vi "Help Queue UI Control.vi"(8 "error In":errorcluster, 11 "CheckPasswordUI.lvclass":refnum<class "CheckPasswordUI.lvclass">) -> (0 "error out":errorcluster)   [LabVIEW 2021, in "CheckPasswordUI.lvclass"]
uses:
  CheckPasswordUI.lvclass
  CheckPasswordUI.lvclass/CheckPasswordUI.ctl
  bc0fb21a-4521-4633-b11b-158f649b6f7e.vi
  <userlib>/John_Lib/Queue_Self/Q-StringToArray_Sushu.vi
  <vilib>/Utility/error.llb/Trim Whitespace.vi
  <userlib>/John_Lib/Queue_Self/Queue_Self.lvlib
panel:
  out "call chain":string[](array[string])
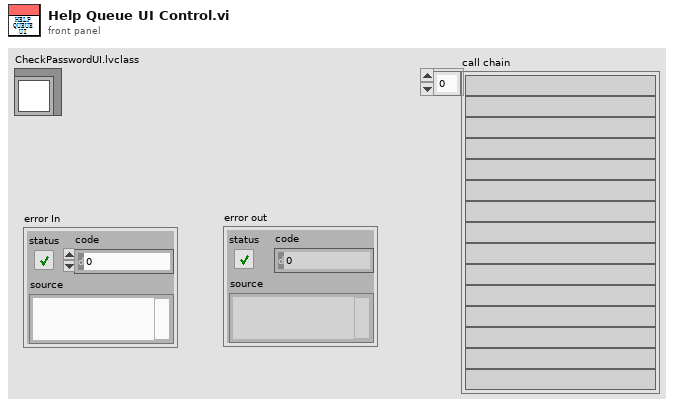
[diagram p1: front panel]
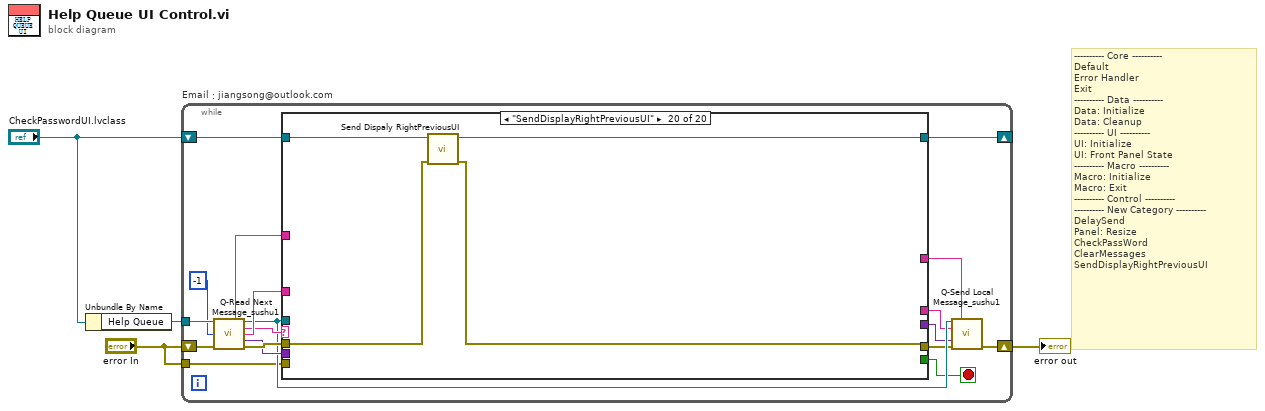
[diagram p0: block diagram]
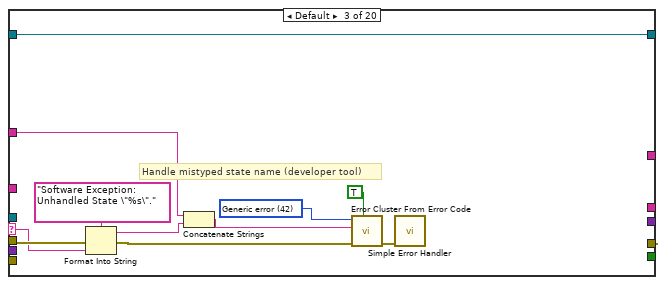
[diagram p4: hidden frame]
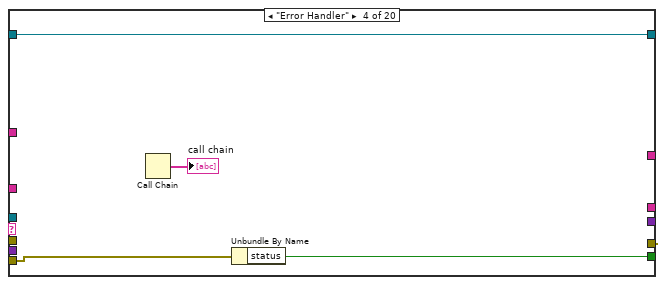
[diagram p5: hidden frame]
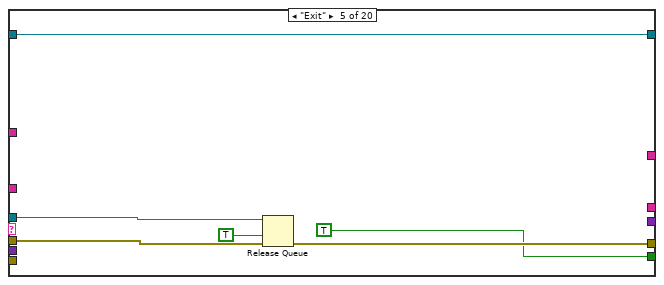
[diagram p6: hidden frame]
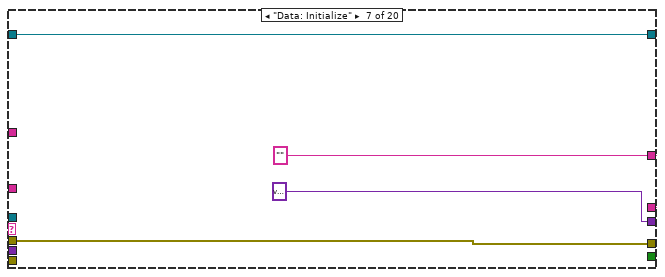
[diagram p8: hidden frame]
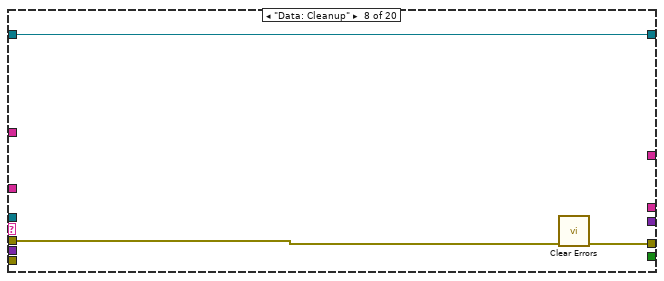
[diagram p9: hidden frame]
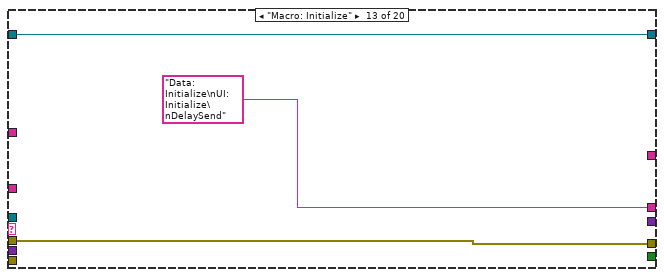
[diagram p14: hidden frame]
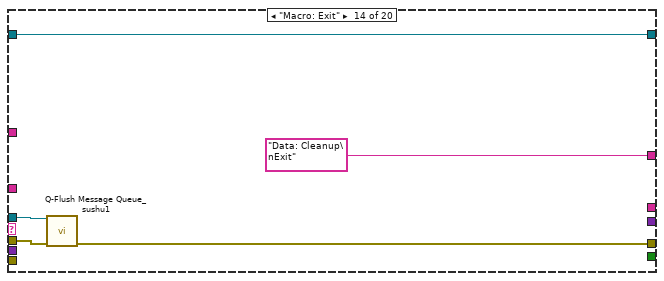
[diagram p15: hidden frame]
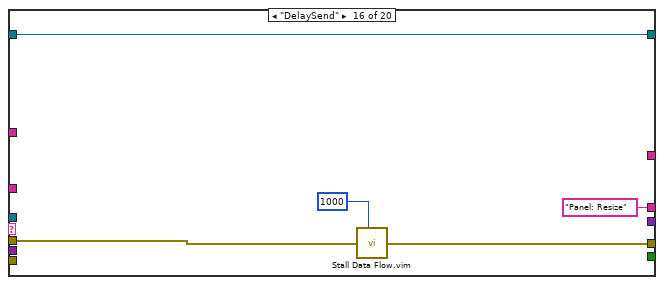
[diagram p17: hidden frame]
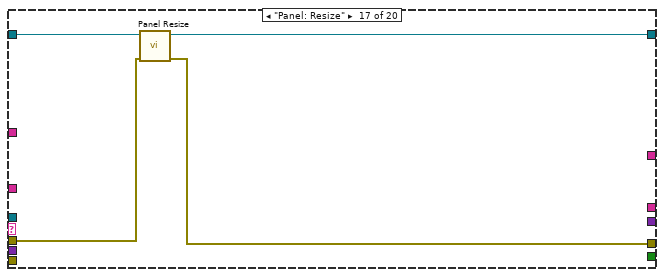
[diagram p18: hidden frame]
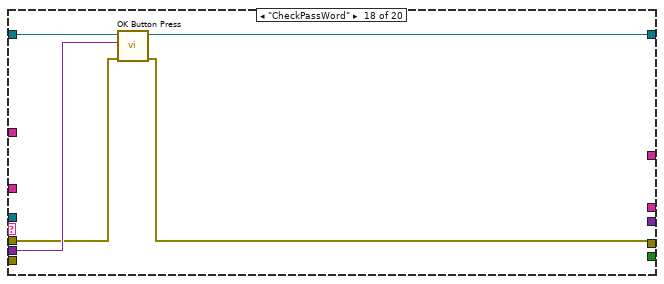
[diagram p19: hidden frame]
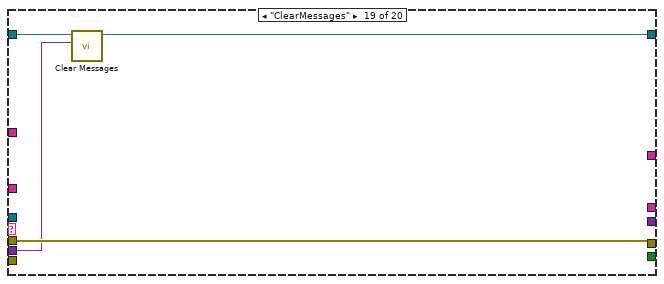
[diagram p20: hidden frame]
diagram:
  # "---------- Core ----------\nDefault\nError Handler\nExit\n---------- Data ----------\nData: Initialize\nData: Cleanup\n---------- UI ----------\nUI: Initialize\nUI: Front Panel State\n---------- Macro ----------\nMacro: Initialize\nMacro: Exit\n---------- Control ----------\n---------- New Category ----------\nDelaySend\nPanel: Resize\nCheckPassWord\nClearMessages\nSendDisplayRightPreviousUI"
  n1 = Unbundle By Name("CheckPasswordUI.lvclass") -> ("Help Queue"=w4:refnum<queue>)
  n2 = while "Email：jiangsong@outlook.com" {
    shift-right: [w11] -> w3
    shift-left: "error In" -> [w7]
    shift-right: [w22] -> _
    shift-left: "CheckPasswordUI.lvclass" -> [w9]
    tunnel: w4 -> [w8]
    tunnel: "error In" -> [w6]
    stop <- w10 stop-if-true
    n3 = call <userlib>:"Q-Read Next Message_sushu1.vi"("queue in"=w8, "timeout (1 ms)"=-1, "error in"=w7) -> ("Previous State + Arguments"=w20:string, "queue out"=w16:refnum<queue>, "Current State"=w17:string, "Arguments"=w19:string, "Data"=w18:variant, "error out"=w21:errorcluster)  [unwired: 6 in, 1 out]
    n4 = case shown="\"SendDisplayRightPreviousUI\"" w17 {
      selector: w17 -> [_ _ w33 _ _ _ _ _ _ _ _ _ _ _ _ _ _ _ _ _]
      tunnel: w16 -> [_ _ _ _ w47 _ _ _ _ _ _ _ _ w72 _ _ _ _ _ _]
      tunnel: w18 -> [_ _ _ _ _ _ _ _ _ _ _ _ _ _ _ _ _ w90 w93 _]
      tunnel: [w23 w26 errorcluster {"status"=FALSE, "code"=0, "source"=""} ("error out") errorcluster {"status"=FALSE, "code"=0, "source"=""} ("error out") w45 w51 w55 w58 w60 w62 w63 w66 w68 w71 w76 w78 w83 w87 w94 w96] -> w15
      tunnel: w21 -> [w23 w26 w34 _ w46 w51 w55 w56 w60 w62 w63 w66 w68 w73 w76 w81 w82 w86 w94 w95]
      tunnel: w9 -> [w24 w25 w28 w43 w49 w50 w54 w57 w59 w61 w64 w65 w69 w74 w75 w80 w84 w88 w91 w97]
      tunnel: [w24 w25 w28 w43 w49 w50 w54 w57 w59 w61 w64 w65 w69 w74 w75 w80 w85 w89 w92 w98] -> w22
      tunnel: w19 -> [_ _ _ _ _ _ _ _ _ _ _ _ _ _ _ _ _ _ _ _]
      tunnel: w20 -> [_ _ w27 _ _ _ _ _ _ _ _ _ _ _ _ _ _ _ _ _]
      tunnel: [_ _ _ _ _ _ w53 _ _ _ _ _ _ "Data: Cleanup\nExit" _ _ _ _ _ _] -> w12
      tunnel: [_ _ _ _ _ _ w53 _ _ _ _ _ "Data: Initialize\nUI: Initialize\nDelaySend" _ _ "Panel: Resize" ("Elements in Front") _ _ _ _] -> w14
      tunnel: [_ _ _ _ _ _ variant ("Data") _ _ _ _ _ _ _ _ _ _ _ _ _] -> w13
      tunnel: [_ _ _ w40 TRUE _ _ _ _ _ _ _ _ _ _ _ _ _ _ _] -> w10
      tunnel: w6 -> [_ _ _ w41 _ _ _ _ _ _ _ _ _ _ _ _ _ _ _ _]
      frame "", "Idle" {
        # "this actor is as the customer UI template\ndon't support message,\nso use queue process Action."
      }
      frame "---------- Core ----------" {
      }
      frame Default {
        w36 = 42 items=["No error", "Argument error", "Memory is full", "Out of zone", "End of file", "File already open", "Generic file I/O error", "File not found", "File permission error", "Disk is full", "Duplicate path", "Too many files open", "System feature not enabled", "Resource file not found", "Cannot add resource", "Resource not found", "Image not found", "Image memory error", "Pen does not exist", "Config type invalid", "Config token not found", "Config parse error", "Config memory error", "Bad external code format", "Bad external code offset", "External code not present", "Null window", "Destroy window error", "Null menu", "Print aborted", "Bad print record", "Print driver error", "Windows error during printing", "Memory error during printing", "Print dialog error", "Generic print error", "Invalid device refnum", "Device not found", "Device parameter error", "Device unit error", "Cannot open device", "Device call aborted", "Generic error", "Cancelled by user", "Object ID too low", "Object ID too high", "Object not in heap", "Unknown heap", "Unknown object (invalid DefProc)", "Unknown object (DefProc not in table)", "Message out of range", "Invalid (null) method", "Unknown message", "Manager call not supported", "Bad address", "Network operation in progress", "Network operation timed out", "Connection is busy", "Network attribute not supported", "Network error", "Address in use", "System out of memory", "Connection aborted", "Connection refused", "Not connected", "Already connected", "Connection closed", "Initialization error (interapplication manager)", "Bad occurrence", "Wait on unbound occurrence handler", "Occurrence queue overflow", "Datalog type conflict", "Unused", "Unrecognized type (interapplication manager)", "Memory corrupt", "Failed to make temporary DLL", "Old CIN version", "Drag socket not found", "Failed to load drop-object", "Failed to register OLE object", "Failed to release OLE object", "Format specifier type mismatch", "Unknown format specifier", "Too few format specifiers", "Too many format specifiers", "Scan failed", "Newer CIN version", "Error converting to variant", "Runtime menu error", "Password tampered", "Variant attribute not found", "Incompatible variant data type", "Event data is not available", "Event Store is not present", "Occurrence is not found", "Event Queue is not created", "Event info is not available", "Refnum passed is NULL", "Error retrieving Class GUID", "Error retrieving CoClass GUID", "Error retrieving TypeLib GUID.", "Bad built application magic bytes.", "Specific driver is different from the specific driver associated with the Logical Name.", "There is no session opened to the class driver.", "Max Error", "MAX - Error with config objects", "MAX - Error loading configuration", "MAX - Group not supported"]
        # "Handle mistyped state name (developer tool)"
        n5 = Format Into String(format string="Software Exception: Unhandled State \"%s\"." ("message"), error in=w34, w33) -> (resulting string=w30:string, error out=w37:errorcluster)  [unwired: 1 in]
        n6 = Concatenate Strings(w27, w30) -> (w29:string)
        n7 = call <vilib>:"Error Cluster From Error Code.vi"("show call chain? (False)"=TRUE, "error in (no error)"=w37, "error message (\"\")"=w29, "error code (0)"=w36) -> ("error out"=w32:errorcluster)  [unwired: 5 in]
        n8 = call <vilib>:"Simple Error Handler.vi"("error in (no error)"=w32) -> ()  [unwired: 4 in, 5 out]
      }
      frame "Error Handler" {
        # "Clear error"
        n9 = Call Chain() -> (call chain=→"call chain":string[])
        n10 = Unbundle By Name(w41) -> ("status"=w40:bool)
      }
      frame "Exit" {
        n11 = Release Queue(queue=w47, force destroy? (F)=TRUE, error in (no error)=w46) -> (error out=w45:errorcluster)  [unwired: 2 out]
      }
      frame "---------- Data ----------" {
      }
      frame "Data: Initialize" {
        w53 = "" ("Elements in Front")
      }
      frame "Data: Cleanup" {
        n12 = call <vilib>:"Clear Errors.vi"("error in (no error)"=w56) -> ("error out"=w58:errorcluster)  [unwired: 5 in, 1 out]
      }
      frame "---------- UI ----------" {
      }
      frame "UI: Initialize" {
      }
      frame "UI: Front Panel State" {
      }
      frame "---------- Macro ----------" {
      }
      frame "Macro: Initialize" {
      }
      frame "Macro: Exit" {
        n13 = call <userlib>:"Q-Flush Message Queue_sushu1.vi"("queue in"=w72, "error in"=w73) -> ("error out"=w71:errorcluster)  [unwired: 11 in, 2 out]
      }
      frame "---------- Control ----------" {
      }
      frame "DelaySend" {
        n14 = call "Stall Data Flow.vim"("value in"=w81, "milliseconds to wait"=u32 1000) -> ("value out"=w78:errorcluster)  [unwired: 1 out]
      }
      frame "Panel: Resize" {
        n15 = call "Panel Resize.vi"("error in (no error)"=w82, "CheckPasswordUI in"=w84) -> ("error out"=w83:errorcluster, "CheckPasswordUI out"=w85:refnum<class "CheckPasswordUI.lvclass">)  [unwired: 8 in]
      }
      frame "CheckPassWord" {
        n16 = call "OK Button Press.vi"("error in (no error)"=w86, "Data"=w90, "CheckPasswordUI in"=w88) -> ("error out"=w87:errorcluster, "CheckPasswordUI out"=w89:refnum<class "CheckPasswordUI.lvclass">)  [unwired: 7 in]
      }
      frame "ClearMessages" {
        n17 = call "Clear Messages.vi"("Data"=w93, "CheckPasswordUI in"=w91) -> ("CheckPasswordUI out"=w92:refnum<class "CheckPasswordUI.lvclass">)  [unwired: 8 in, 1 out]
      }
      frame "SendDisplayRightPreviousUI" {
        n18 = call "Send Dispaly RightPreviousUI.vi"("error in (no error)"=w95, "CheckPasswordUI in"=w97) -> ("error out"=w96:errorcluster, "CheckPasswordUI out"=w98:refnum<class "CheckPasswordUI.lvclass">)  [unwired: 8 in]
      }
    }
    n19 = call <userlib>:"Q-Send Local Message_sushu1.vi"("queue in"=w16, "Elements in Front"=w12, "Elements at Back"=w14, "message value"=w13, "error in"=w15) -> ("error out"=w11:errorcluster)  [unwired: 8 in, 2 out]
  }
  "error out" <- w3
